vi "Main (old).vi"() -> ()   [LabVIEW 2018]
uses:
  <extravilib>/ChannelInstances/Stream-a[.](t'SR Cluster.ctl').lvlib
  Type Defs/SR Status.ctl
  Type Defs/SR Cluster.ctl
panel:
  in  "Labels":string="SR #                   SR Status                          SR Type              Summary                                                                           Last Updated      Service Level     Days Open   Creation Date                   "
  in  "Refresh SRs":bool
  in  "Add SR":bool
  in  "Stop":bool
  in  "Sorting":T1(ring)
  out "SR List":T2[](array[typedef]) {"Creation Date" format="%<%x>T"; "Last Updated" format="%<%x>T"; "Days Open" format="%#.1f"}
  in  "Filter Cluster":T4={"Show Resolved"=TRUE, "Show Potentially Resolved"=TRUE, "Show Passoffs"=TRUE, "Show In Collab"=TRUE}
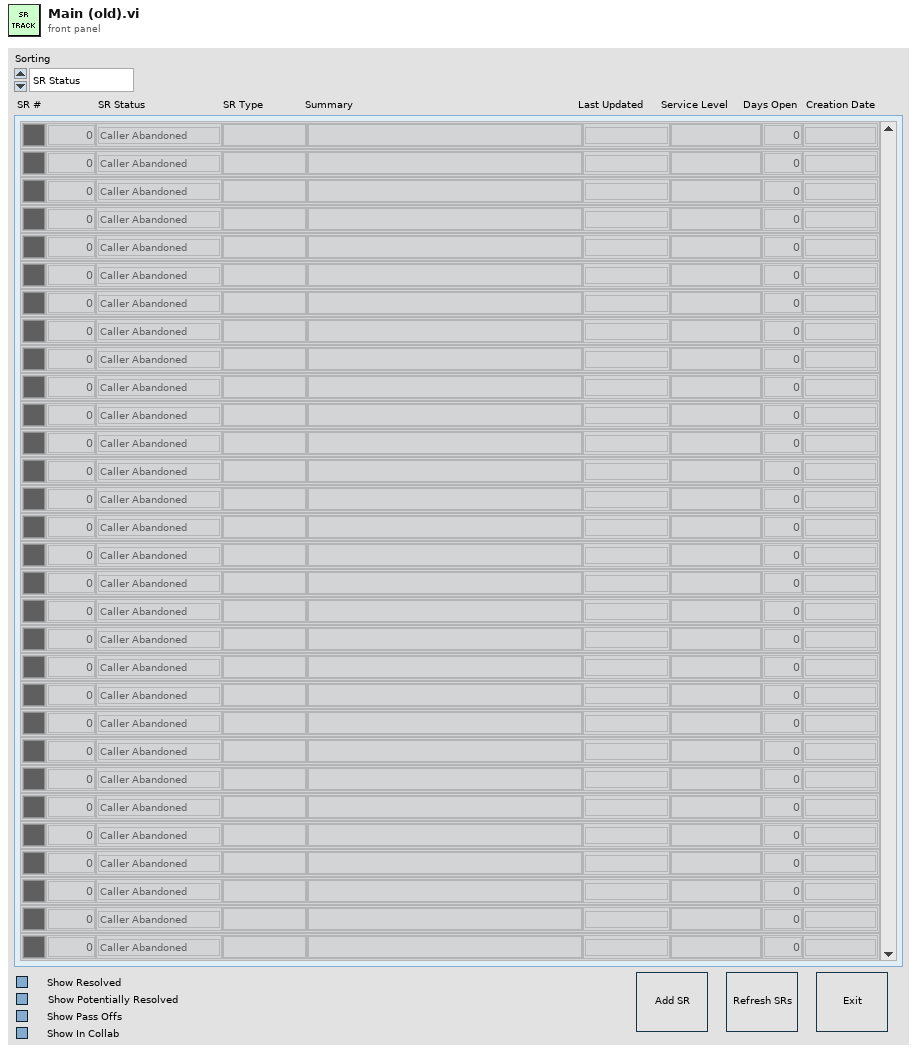
[diagram p1: front panel]
types:
  T1 = enum16{"SR Status", "Most Recent", "SR Type", "SR Number"}
  T2 = typedef "SR Cluster.ctl" = cluster{"Color":u32, "SR Number":i32, "SR Status":T3, "SR Type":string, "Summary":string, "Last Updated":timestamp, "Service Level":string, "Days Open":dbl, "Creation Date":timestamp}
  T3 = typedef "SR Status.ctl" = enum16{"Caller Abandoned", "Created in Error", "Expired", "Forum Resolved AE", "Forum Resolved Customer", "IN WORK", "IN WORK Collab with AES", "IN WORK Collab with PSE", "IN WORK Collab with SE", "IN WORK Customer Added Note", "IN WORK Escalation", "IN WORK Wait on Customer", "Open", "Potentially Resolved", "Presumed Resolved", "RMA Approved for Return", "Resolved", "Passed Off"}
  T4 = cluster{"Show Resolved":bool, "Show Potentially Resolved":bool, "Show Passoffs":bool, "Show In Collab":bool}
  T5 = enum8{"Enabled", "Disabled", "Disabled and Grayed Out"}
  T6 = typedef "Stream-a[.](t'SR Cluster.ctl').lvlib/)Channel.ctl" = refnum<queue>
  T7 = enum32{"invalid app kind", "Development System", "Run Time System", "Student Edition", "Embedded LabVIEW", "Evaluation", "Custom"}
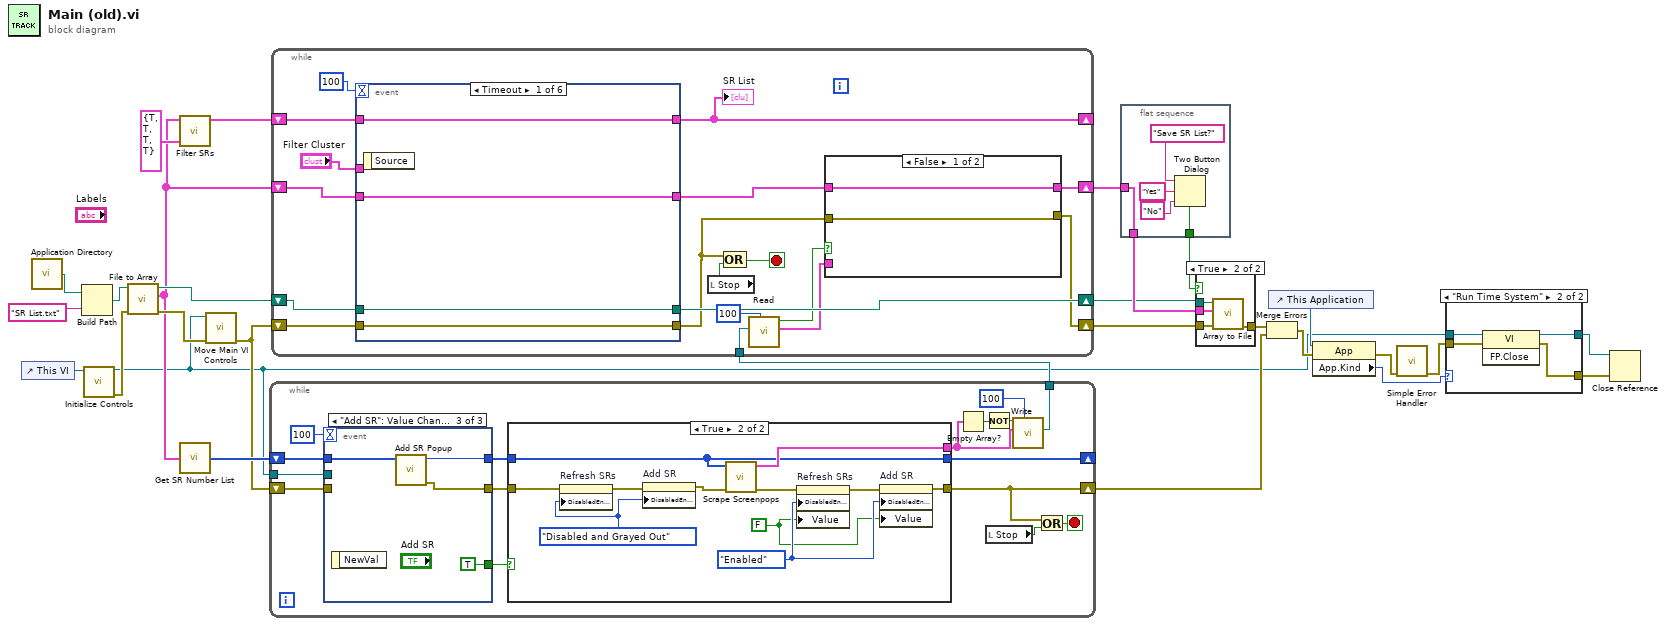
[diagram p0: block diagram]
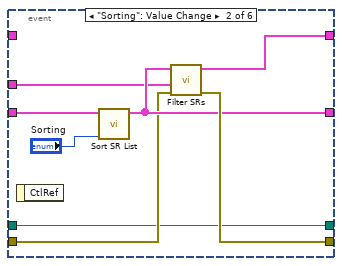
[diagram p2: hidden frame]
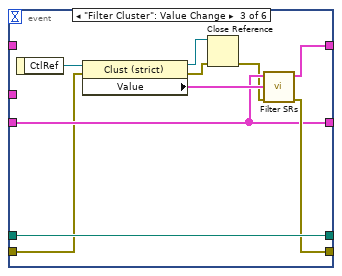
[diagram p3: hidden frame]
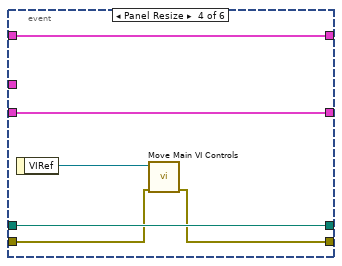
[diagram p4: hidden frame]
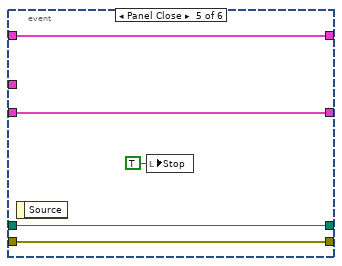
[diagram p5: hidden frame]
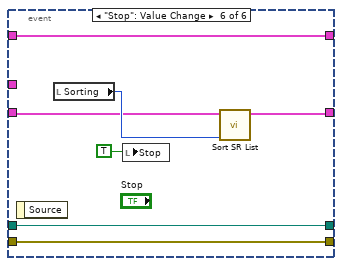
[diagram p6: hidden frame]
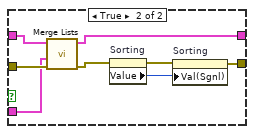
[diagram p7: hidden frame]
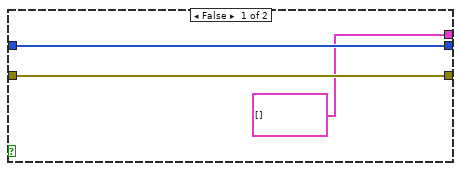
[diagram p8: hidden frame]
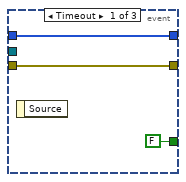
[diagram p9: hidden frame]
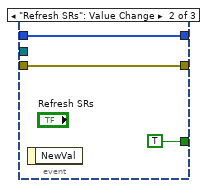
[diagram p10: hidden frame]
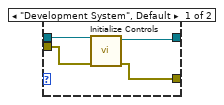
[diagram p12: hidden frame]
diagram:
  n1 = control-ref of="This VI"() -> (w3:refnum<vi>)
  n2 = call <vilib>:"Application Directory.vi"() -> ("Application Directory"=w8:path)
  n3 = Build Path(base path=w8, name or relative path="SR List.txt") -> (appended path=w26:path)
  n4 = call "Initialize Controls.vi"("VI refnum in"=w3) -> ("error out"=w4:errorcluster, "VI refnum out"=w1:refnum<vi>)  [unwired: 9 in]
  n5 = call "File to Array.vi"("error in"=w4, "file path in"=w26) -> ("error out"=w25:errorcluster, "list out"=w18:T2[], "file path out"=w28:path)  [unwired: 7 in]
  n6 = call "Filter SRs.vi"("Filter Cluster"=T4 {"Show Resolved"=TRUE, "Show Potentially Resolved"=TRUE, "Show Passoffs"=TRUE, "Show In Collab"=TRUE} ("Filter Cluster 2"), "list in"=w18) -> ("list out"=w20:T2[])  [unwired: 8 in, 1 out]
  n7 = call "Get SR Number List.vi"("list in"=w18) -> ("SR number array out"=w17:i32[])  [unwired: 4 in]
  n8 = call "Move Main VI Controls.vi"("error in"=w25, "VIRef in"=w1) -> ("error out"=w16:errorcluster)  [unwired: 9 in]
  n9 = while {
    shift-right: [w32] -> _
    shift-left: w17 -> [w43]
    shift-right: [w35] -> w5
    shift-left: w16 -> [w42]
    tunnel: [w38] -> w15
    tunnel: w1 -> [w29]
    stop <- w41 stop-if-true
    n10 = event shown="[2] \"Add SR\": Value Change" {
      selector: _ -> [_ _ _]
      dyn-events: _ -> [_ _ _]
      timeout: 100 -> [_ _ _]
      tunnel: w43 -> [w60 w64 w68]
      tunnel: w42 -> [w61 w63 _]
      tunnel: [w61 w63 w65] -> w34
      tunnel: [w60 w64 w67] -> w33
      tunnel: [FALSE TRUE TRUE] -> w36
      tunnel: w29 -> [_ _ _]
      event Timeout {
        n11 = event-data() -> ()  [unwired: 1 in, 1 out]
      }
      event "Refresh SRs": Value Change {
        n12 = event-data() -> ()  [unwired: 1 in, 1 out]
      }
      event "Add SR": Value Change {
        n13 = event-data() -> ()  [unwired: 1 in, 1 out]
        n14 = call "Add SR Popup.vi"(11:w68) -> ("error out"=w65:errorcluster, "SR out"=w67:i32)  [unwired: 8 in, 1 out]
      }
    }
    n15 = case shown="True" w36 {
      tunnel: [w46 w53] -> w35
      tunnel: w34 -> [w46 w48]
      tunnel: [w47 w57] -> w32
      tunnel: w33 -> [w47 w57]
      tunnel: [T2[] [] ("sr clusters out") w58] -> w30
      frame False {
      }
      frame True {
        w50 = T5."Disabled and Grayed Out" ("Disabled")
        w52 = FALSE ("Refresh SRs")
        w56 = T5."Enabled" ("Disabled")
        n16 = property on="Refresh SRs" class="Bool (strict)"(error in=w48, "DisabledEnum"=w50) -> (error out=w51:errorcluster)  [unwired: 1 in, 1 out]
        n17 = property on="Add SR" class="Bool (strict)"(error in=w51, "DisabledEnum"=w50) -> (error out=w49:errorcluster)  [unwired: 1 in, 1 out]
        n18 = call "Scrape Screenpops.vi"("error in"=w49, "SR number list in"=w57) -> ("error out"=w55:errorcluster, "sr clusters out"=w58:T2[])  [unwired: 8 in]
        n19 = property on="Refresh SRs" class="Bool (strict)"(error in=w55, "DisabledEnum"=w56, "Value"=w52) -> (error out=w54:errorcluster)  [unwired: 1 in, 1 out]
        n20 = property on="Add SR" class="Bool (strict)"(error in=w54, "DisabledEnum"=w56, "Value"=w52) -> (error out=w53:errorcluster)  [unwired: 1 in, 1 out]
      }
    }
    n21 = Empty Array?(array=w30) -> (empty?=w40:bool)
    n22 = Not(x=w40) -> (.not. x?=w39:bool)
    n23 = local read "Stop"() -> (w31:bool)
    n24 = call <extravilib>:"Write.vi"("timeout in ms (-1)"=100, "element"=w30, "element valid? (T)"=w39) -> ("channel"=w38:T6)  [unwired: 6 in, 2 out]
    n25 = Or(x=w35, y=w31) -> (x .or. y?=w41:bool)
  }
  n26 = while {
    shift-right: [w84] -> w2
    shift-left: w28 -> [w69]
    shift-right: [w71] -> w13
    shift-left: w16 -> [w70]
    shift-right: [w76] -> w10
    shift-left: w18 -> [w85]
    shift-right: [w73] -> _
    shift-left: w20 -> [w82]
    tunnel: w15 -> [w80]
    stop <- w83 stop-if-true
    n27 = event shown="[0] Timeout" {
      selector: _ -> [_ _ _ _ _ _]
      dyn-events: _ -> [_ _ _ _ _ _]
      timeout: 100 -> [_ _ _ _ _ _]
      tunnel: [w90 w91 w107 w114 w119 w125] -> w84
      tunnel: w69 -> [w90 w91 w107 w114 w119 w125]
      tunnel: [w87 w97 w106 w111 w118 w124] -> w74
      tunnel: w70 -> [w87 w93 w102 w112 w118 w124]
      tunnel: w85 -> [w89 w98 w105 w113 w117 w120]
      tunnel: [w89 w96 w105 w113 w117 w122] -> w75
      tunnel: [w88 w92 w104 w109 w116 w123] -> w73
      tunnel: w82 -> [w88 _ _ w109 w116 w123]
      tunnel: "Filter Cluster" -> [_ w94 _ _ _ _]
      event Timeout {
        n28 = event-data() -> ()  [unwired: 1 in, 1 out]
      }
      event "Sorting": Value Change {
        n29 = event-data() -> ()  [unwired: 1 in, 1 out]
        n30 = call "Sort SR List.vi"("Sorting"="Sorting", "list in"=w98) -> ("list out"=w96:T2[])  [unwired: 9 in]
        n31 = call "Filter SRs.vi"("error in"=w93, "Filter Cluster"=w94, "list in"=w96) -> ("error out"=w97:errorcluster, "list out"=w92:T2[])  [unwired: 7 in]
      }
      event "Filter Cluster": Value Change {
        n32 = event-data() -> ("CtlRef"=w99:refnum<vi>)  [unwired: 1 in]
        n33 = property class="Clust (strict)"(reference=w99, error in=w102) -> (reference out=w101:refnum<vi>, error out=w100:errorcluster, "Value"=w108:T4)
        n34 = Close Reference(reference=w101, error in (no error)=w100) -> (error out=w103:errorcluster)
        n35 = call "Filter SRs.vi"("error in"=w103, "Filter Cluster"=w108, "list in"=w105) -> ("error out"=w106:errorcluster, "list out"=w104:T2[])  [unwired: 7 in]
      }
      event Panel Resize {
        n36 = event-data() -> ("VIRef"=w110:refnum<vi>)  [unwired: 1 in]
        n37 = call "Move Main VI Controls.vi"("error in"=w112, "VIRef in"=w110) -> ("error out"=w111:errorcluster)  [unwired: 9 in]
      }
      event Panel Close {
        n38 = event-data() -> ()  [unwired: 1 in, 1 out]
        n39 = local write "Stop"(TRUE ("Stop")) -> ()
      }
      event "Stop": Value Change {
        n40 = event-data() -> ()  [unwired: 1 in, 1 out]
        n41 = local read "Sorting"() -> (w121:T1)
        n42 = local write "Stop"(TRUE ("Stop")) -> ()
        n43 = call "Sort SR List.vi"("Sorting"=w121, "list in"=w120) -> ("list out"=w122:T2[])  [unwired: 9 in]
      }
    }
    "SR List" <- w73
    n44 = local read "Stop"() -> (w81:bool)
    n45 = Compound Arithmetic op=OR(w74, w81) -> (w83:bool)
    n46 = call <extravilib>:"Read.vi"("timeout in ms (-1)"=100, "channel"=w80) -> ("element"=w78:T2[], "element valid?"=w77:bool)  [unwired: 5 in, 3 out]
    n47 = case shown="False" w77 {
      tunnel: w78 -> [_ w134]
      tunnel: [w128 w133] -> w76
      tunnel: w75 -> [w128 w135]
      tunnel: w74 -> [w127 w136]
      tunnel: [w127 w132] -> w71
      frame False {
      }
      frame True {
        n48 = call "Merge Lists.vi"("error in"=w136, "new list in"=w134, "list in"=w135) -> ("error out"=w129:errorcluster, "list out"=w133:T2[])  [unwired: 7 in]
        n49 = property on="Sorting" class="Enum (strict)"(error in=w129) -> (error out=w130:errorcluster, "Value"=w131:T1)  [unwired: 1 in, 1 out]
        n50 = property on="Sorting" class="Enum (strict)"(error in=w130, "Val(Sgnl)"=w131) -> (error out=w132:errorcluster)  [unwired: 1 in, 1 out]
      }
    }
  }
  n51 = flat-sequence {
    tunnel: [w141] -> w11
    tunnel: [w137] -> w9
    tunnel: w10 -> [w137]
    frame #0 {
      n52 = Two Button Dialog(message="Save SR List?", 1:"No" ("F button name (\"Cancel\")"), 2:"Yes" ("T button name (\"OK\")")) -> (T button?=w141:bool)
    }
  }
  n53 = case shown="True" w11 {
    tunnel: w13 -> [w142 w146]
    tunnel: [w142 w145] -> w12
    tunnel: w2 -> [_ w144]
    tunnel: w9 -> [_ w143]
    frame False {
    }
    frame True {
      n54 = call "Array to File.vi"("error in"=w146, "array in"=w143, "file path in"=w144) -> ("error out"=w145:errorcluster)  [unwired: 7 in, 1 out]
    }
  }
  n55 = Merge Errors(w12, w5) -> (w14:errorcluster)
  n56 = control-ref of="This Application"() -> (w24:refnum<vi>)
  n57 = property class="App"(reference=w24, error in=w14) -> (error out=w21:errorcluster, "App.Kind"=w22:T7)  [unwired: 1 out]
  n58 = call <vilib>:"Simple Error Handler.vi"("error in (no error)"=w21) -> ("error out"=w23:errorcluster)  [unwired: 4 in, 4 out]
  n59 = case shown="\"Run Time System\"" w22 {
    tunnel: w23 -> [w149 w154]
    tunnel: w1 -> [w150 w153]
    tunnel: [w147 w152] -> w7
    tunnel: [w148 w151] -> w6
    frame "Development System", Default {
      n60 = call "Initialize Controls.vi"("error in"=w149, "VI refnum in"=w150) -> ("error out"=w148:errorcluster, "VI refnum out"=w147:refnum<vi>)  [unwired: 8 in]
    }
    frame "Run Time System" {
      n61 = invoke class="VI" method="FP.Close"(reference=w153, error in=w154) -> (reference out=w152:refnum<vi>, error out=w151:errorcluster)  [unwired: 1 in, 1 out]
    }
  }
  n62 = Close Reference(reference=w7, error in (no error)=w6) -> ()  [unwired: 1 out]
